vi "GEOM_ReadOverrideWCSFile.vi"(10 "Path":path=path "/home/bonati/panview_current/fpas/_echelle/config/GEOM_OVERRIDE_WCS.tpl") -> ()   [LabVIEW 2016]
uses:
  GEOM_VAR_action.ctl
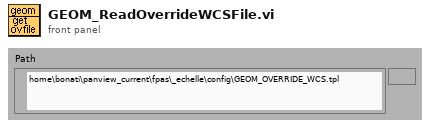
[diagram p1: front panel]
types:
  T1 = typedef "GEOM_VAR_action.ctl" = enum16{"read", "write"}
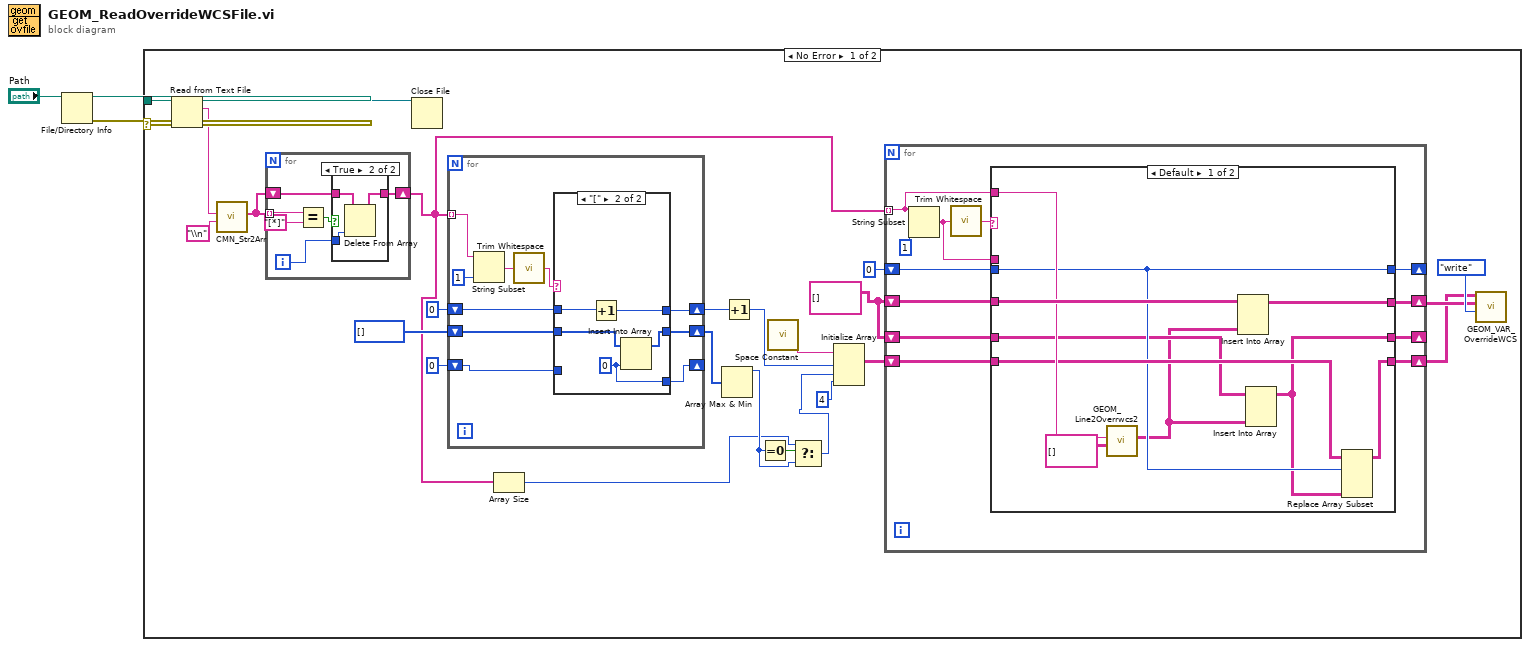
[diagram p0: block diagram]
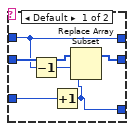
[diagram p3: hidden frame]
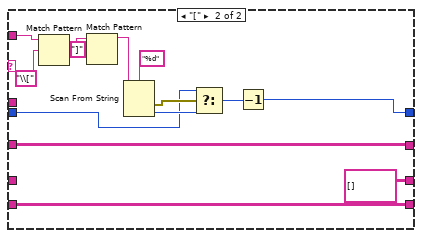
[diagram p4: hidden frame]
diagram:
  n1 = File/Directory Info(path="Path") -> (path out=w1:path, error out=w2:errorcluster)  [unwired: 1 in, 5 out]
  n2 = case shown="No Error" w2 {
    tunnel: w1 -> [w27 _]
    frame No Error {
      w6 = string[][] [] ("out")
      n3 = Read from Text File(file (use dialog)=w27) -> (refnum out=w26:refnum<file>, text=w23:string)  [unwired: 1 in, 4 out]
      n4 = call "CMN_Str2Arr.vi"("separator"="\\n", "string in"=w23) -> ("Array out"=w5:string[])  [unwired: 2 in, 7 out]
      n5 = for {
        tunnel: w5 -> [w33] mode=indexing
        shift-right: [w29] -> w4
        shift-left: w5 -> [w30]
        i -> [w28]
        n6 = Equal?(x=w33, y="[*]") -> (x = y?=w31:bool)
        n7 = case shown="True" w31 {
          tunnel: w30 -> [w34 w37]
          tunnel: [w34 w35] -> w29
          tunnel: w28 -> [_ w36]
          frame False {
          }
          frame True {
            n8 = Delete From Array(array=w37, index=w36) -> (array with subset deleted=w35:string[])  [unwired: 1 in, 1 out]
          }
        }
      }
      n9 = Close File(refnum=w26) -> ()  [unwired: 1 in, 2 out]
      n10 = for {
        tunnel: w4 -> [w46] mode=indexing
        shift-right: [w43] -> w12
        shift-left: 0 -> [w42]
        shift-right: [w40] -> w14
        shift-left: i32[] [] -> [w41]
        shift-right: [w39] -> _
        shift-left: 0 ("new element/subarray") -> [w38]
        n11 = String Subset(string=w46, length (rest)=1 ("length (rest)")) -> (substring=w47:string)  [unwired: 1 out]
        n12 = call <vilib>:"Trim Whitespace.vi"("string"=w47) -> ("trimmed string"=w44:string)  [unwired: 1 in]
        n13 = case shown="\"[\"" w44 {
          tunnel: [w49 w57] -> w43
          tunnel: w42 -> [w49 w58]
          tunnel: w41 -> [w52 w55]
          tunnel: [w50 w56] -> w40
          tunnel: [w51 w54] -> w39
          tunnel: w38 -> [w53 _]
          frame Default {
            n14 = Decrement(x=w49) -> (x-1=w48:i32)
            n15 = Increment(x=w53) -> (x+1=w51:i32)
            n16 = Replace Array Subset(array=w52, new element=w51, index=w48) -> (w50:i32[])
          }
          frame "[" {
            w54 = 0 ("new element/subarray")
            n17 = Increment(x=w58) -> (x+1=w57:i32)
            n18 = Insert Into Array(array=w55, new element=w54) -> (w56:i32[])  [unwired: 1 in]
          }
        }
      }
      n19 = Array Size(array=w4) -> (size(s)=w8:i32)
      n20 = Array Max & Min(array=w14) -> (max value=w9:i32)  [unwired: 3 out]
      n21 = Increment(x=w12) -> (x+1=w11:i32)
      n22 = Equal To 0?(x=w9) -> (x = 0?=w10:bool)
      n23 = call <vilib>:"Space Constant.vi"() -> ("String"=w13:string)
      n24 = Select(t=w8, s=w10, f=w9) -> (s? t:f=w7:i32)
      n25 = Initialize Array(w13, w11, w7, 4 ("dimension size")) -> (w19:string[][][])
      n26 = for {
        tunnel: w4 -> [w67] mode=indexing
        shift-right: [w65] -> w22
        shift-left: w6 -> [w66]
        shift-right: [w63] -> w21
        shift-left: w19 -> [w64]
        shift-right: [w62] -> _
        shift-left: 0 -> [w61]
        shift-right: [w60] -> _
        shift-left: w6 -> [w59]
        n27 = String Subset(string=w67, length (rest)=1 ("length (rest)")) -> (substring=w68:string)  [unwired: 1 out]
        n28 = call <vilib>:"Trim Whitespace.vi"("string"=w68) -> ("trimmed string"=w69:string)  [unwired: 1 in]
        n29 = case shown="Default" w69 {
          tunnel: w68 -> [_ _]
          tunnel: w67 -> [w79 w93]
          tunnel: w66 -> [w80 w94]
          tunnel: [w74 w94] -> w65
          tunnel: w64 -> [w76 w83]
          tunnel: [w77 w83] -> w63
          tunnel: [w75 w82] -> w62
          tunnel: w61 -> [w75 w88]
          tunnel: [w71 string[][] [] ("out")] -> w60
          tunnel: w59 -> [w73 _]
          frame Default {
            n30 = call "GEOM_Line2Overrwcs2.vi"("curr arr"=string[][] [], "extension data"=w79) -> ("out"=w72:string[][])  [unwired: 9 out]
            n31 = Insert Into Array(array=w80, new element=w72) -> (w74:string[][])  [unwired: 2 in]
            n32 = Insert Into Array(array=w73, new element=w72) -> (w71:string[][])  [unwired: 2 in]
            n33 = Replace Array Subset(array=w76, new element=w71, index (dim 0)=w75) -> (w77:string[][][])  [unwired: 2 in]
          }
          frame "[" {
            n34 = Match Pattern(string=w93, regular expression="\\[") -> (after substring=w86:string)  [unwired: 4 out]
            n35 = Match Pattern(string=w86, regular expression="]") -> (before substring=w84:string)  [unwired: 4 out]
            n36 = Scan From String(format string="%d", input string=w84) -> (error out=w90:errorcluster, output 1=w89:i32)  [unwired: 2 in, 3 out]
            n37 = Select(t=w88, s=w90, f=w89) -> (s? t:f=w87:i32)
            n38 = Decrement(x=w87) -> (x-1=w82:i32)
          }
        }
      }
      n39 = call "GEOM_VAR_OverrideWCS.vi"("Action"=GEOM_VAR_action."write", "override headers"=w22, "override headers mext"=w21) -> ()  [unwired: 9 out]
    }
    frame Error {
    }
  }
